vi "SLL DE Generate Custom Error.vi"(6 "No of Callers to add":i32=1, 7 "Case Name":string, 8 "error in":errorcluster, 10 "Error Code (0)":i32, 11 "Error? (T)":bool=TRUE) -> (0 "error out":errorcluster)   [LabVIEW 2013]
doc: "Creates the error cluster given the error status and code.It also adds the specified no of caller vi names and the message to the source.\n\n<B>Note : </B> Custom Error code & error description should be added in the Error code file and it should be attached during building Application (EXE)\n\nCopyright © 2006, Soliton Technologies. All rights reserved."
panel:
  # "Inputs"
  # "Outputs"
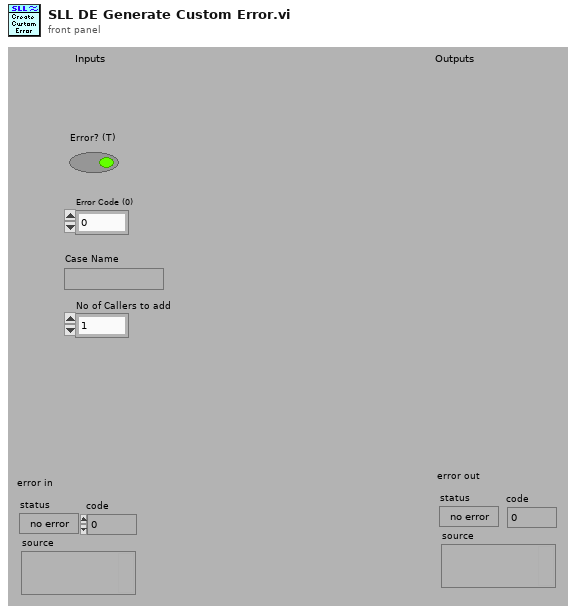
[diagram p1: front panel]
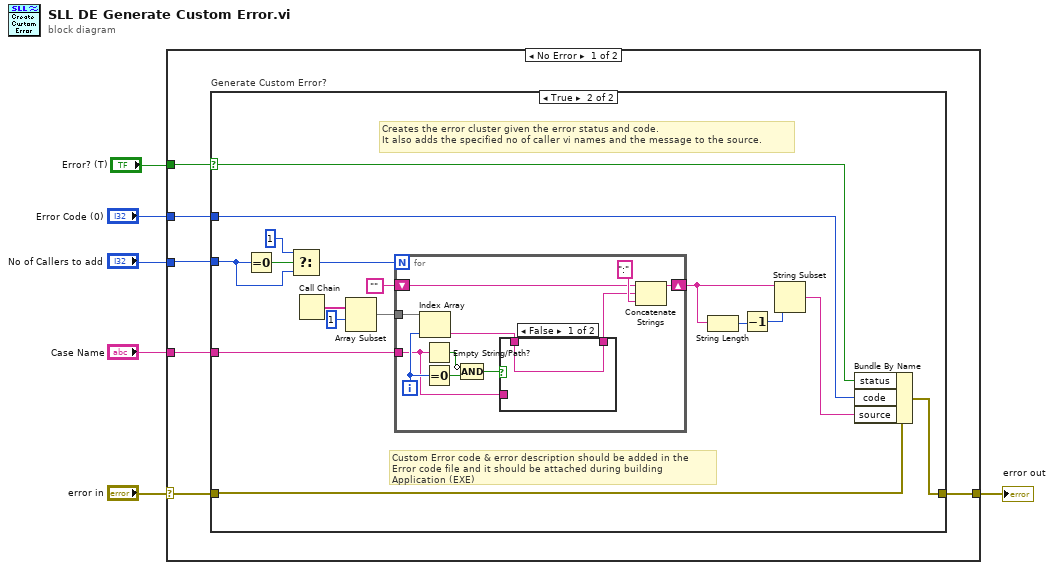
[diagram p0: block diagram]
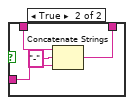
[diagram p3: hidden frame]
diagram:
  n1 = case shown="No Error" "error in" {
    selector: "error in" -> [w11 w47]
    tunnel: [w12 w47] -> w6
    tunnel: "Error? (T)" -> [w7 _]
    tunnel: "No of Callers to add" -> [w9 _]
    tunnel: "Error Code (0)" -> [w10 _]
    tunnel: "Case Name" -> [w8 _]
    frame No Error {
      n2 = case "Generate Custom Error?" shown="True" w7 {
        selector: w7 -> [_ w18]
        tunnel: [w13 w30] -> w12
        tunnel: w11 -> [w13 w29]
        tunnel: w10 -> [_ w24]
        tunnel: w9 -> [_ w21]
        tunnel: w8 -> [_ w19]
        frame False {
          # "Passes the incoming error cluster if there is no custom error in input stage."
        }
        frame True {
          # "Custom Error code & error description should be added in the Error code file and it should be attached during building Application (EXE)"
          # "Creates the error cluster given the error status and code.\nIt also adds the specified no of caller vi names and the message to the source."
          n3 = Equal To 0?(x=w21) -> (x = 0?=w23:bool)
          n4 = Select(t=1 ("Array Index"), s=w23, f=w21) -> (s? t:f=w20:i32)
          n5 = Call Chain() -> (call chain=w28:string[])
          n6 = Array Subset(array=w28, index=1 ("Array Index")) -> (w26:string[])  [unwired: 1 in]
          n7 = for {
            N: w20 -> [_]
            tunnel: w26 -> [w41]
            shift-right: [w38] -> w17
            shift-left: "" -> [w39]
            tunnel: w19 -> [w33]
            i -> [w37]
            n8 = Index Array(array=w41, index=w37) -> (element=w31:string)
            n9 = Empty String/Path?(string/path=w33) -> (empty?=w35:bool)
            n10 = Equal To 0?(x=w37) -> (x = 0?=w36:bool)
            n11 = Compound Arithmetic op=AND(invert w35, w36) -> (w34:bool)
            n12 = case shown="False" w34 {
              tunnel: w33 -> [_ w45]
              tunnel: w31 -> [w42 w46]
              tunnel: [w42 w43] -> w32
              frame False {
              }
              frame True {
                n13 = Concatenate Strings(w46, "-" ("string"), w45) -> (w43:string)
              }
            }
            n14 = Concatenate Strings(w39, w32, ":") -> (w38:string)
          }
          n15 = String Length(string=w17) -> (length=w16:i32)
          n16 = Decrement(x=w16) -> (x-1=w15:i32)
          n17 = String Subset(string=w17, length (rest)=w15) -> (substring=w14:string)  [unwired: 1 in]
          n18 = Bundle By Name(cluster=w29, "status"=w18, "code"=w24, "source"=w14) -> (w30:errorcluster)
        }
      }
    }
    frame Error {
      # "Passes the error if there is error in input stage."
    }
  }
  "error out" <- w6
